vi "Print Report.vi"(2 "error in":errorcluster, 3 "Language":T1, 4 "Initial Path":path) -> (0 "error IO":errorcluster, 1 "Message":string)   [LabVIEW 2015]
uses:
  CustomControl/Lang_Control.ctl
  <vilib>/Utility/NIReport.llb/NI_report.lvclass
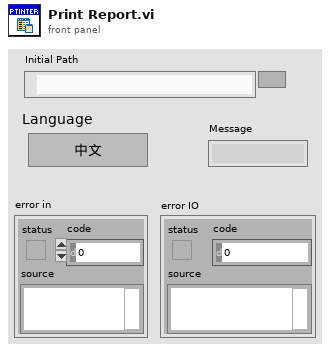
[diagram p1: front panel]
types:
  T1 = typedef "Lang_Control.ctl" = enum16{"中文", "English"}
  T2 = enum16{"maximized", "minimized", "normal", "no change"}
  T3 = enum16{"Standard Report", "HTML", "Word", "Excel"}
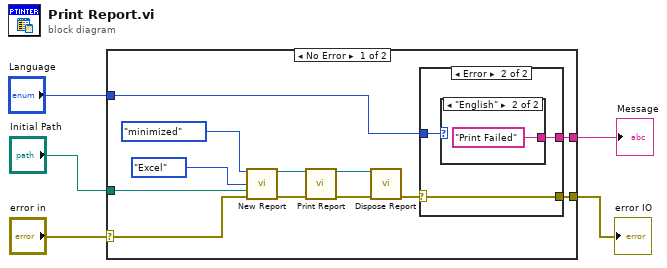
[diagram p0: block diagram]
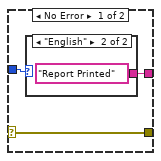
[diagram p2: hidden frame]
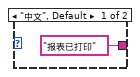
[diagram p3: hidden frame]
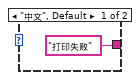
[diagram p4: hidden frame]
diagram:
  n1 = case shown="No Error" "error in" {
    selector: "error in" -> [w6 w28]
    tunnel: [w10 w28] -> w4
    tunnel: [w9 _] -> w3
    tunnel: "Language" -> [w8 _]
    tunnel: "Initial Path" -> [w7 _]
    frame No Error {
      n2 = call <vilib>:"New Report.vi"("window state (normal)"=T2."minimized", "report type"=T3."Excel", "template (empty)"=w7, "error in (no error)"=w6) -> ("report out"=w17:refnum<class "NI_report.lvclass">, "error out"=w16:errorcluster)  [unwired: 10 in]
      n3 = call-dynamic "Print Report.vi"("report in"=w17, "error in (no error)"=w16) -> ("report out"=w15:refnum<class "NI_report.lvclass">, "error out"=w14:errorcluster)  [unwired: 12 in]
      n4 = call-dynamic "Dispose Report.vi"("report in"=w15, "error in (no error)"=w14) -> ("error out"=w11:errorcluster)  [unwired: 13 in]
      n5 = case shown="Error" w11 {
        selector: w11 -> [w20 w23]
        tunnel: [w20 w23] -> w10
        tunnel: [w19 w25] -> w9
        tunnel: w8 -> [w18 w24]
        frame No Error {
          n6 = case shown="\"English\"" w18 {
            tunnel: ["报表已打印" "Report Printed"] -> w19
            frame "中文", Default {
            }
            frame "English" {
            }
          }
        }
        frame Error {
          n7 = case shown="\"English\"" w24 {
            tunnel: ["打印失败" "Print Failed"] -> w25
            frame "中文", Default {
            }
            frame "English" {
            }
          }
        }
      }
    }
    frame Error {
    }
  }
  "error IO" <- w4
  "Message" <- w3
